vi "Transition Matrices_v1.vi"(6 "alpha":dbl, 8 "Tassign":dbl[](array[numeric])=[3.0, 4.0], 9 "theta":dbl=-0.6435 format="%#_13g", 10 "Rassign":dbl=1.0 format="%#_13g", 11 "R0":dbl) -> (1 "Translation Vector":dbl[](array[numeric]), 3 "Rotation Matrix":dbl[][](array[numeric]))   [LabVIEW 2010]
doc: "This file calculates the index-dependent rotation matrix and translation vector.\nReye is the eye radius, Rassign is the assigned radius, Tassign is the assigned translation vector.\nalpha is the scaling time-dependent parameter varys from 0 to 1."
uses:
  <vilib>/Analysis/NI_AALPro.lvlib
  <vilib>/Analysis/_algsub.llb/Real Vector Norm.vi
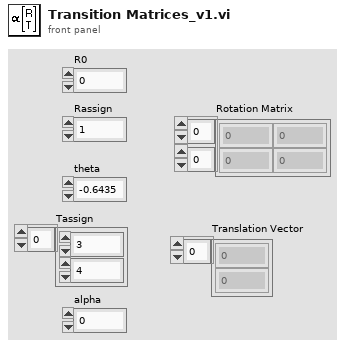
[diagram p1: front panel]
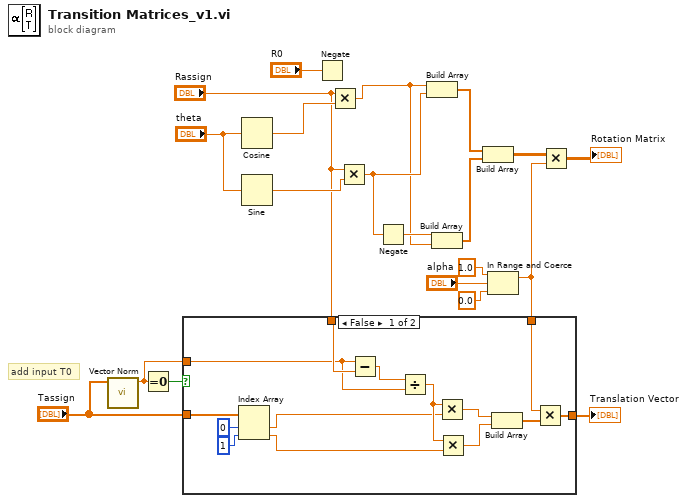
[diagram p0: block diagram]
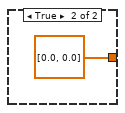
[diagram p2: hidden frame]
diagram:
  # "add input T0"
  n1 = call-poly <vilib>:"Vector Norm.vi"("Input Vector"="Tassign") -> ("norm"=w6:dbl)  [unwired: 9 in, 1 out]
  n2 = Equal To 0?(x=w6) -> (x = 0?=w4:bool)
  n3 = Cosine(x="theta") -> (cos(x)=w20:dbl)
  n4 = Sine(x="theta") -> (sin(x)=w19:dbl)
  n5 = Negate(x="R0") -> ()  [unwired: 1 out]
  n6 = Multiply(x="Rassign", y=w20) -> (x*y=w1:dbl)
  n7 = Multiply(x="Rassign", y=w19) -> (x*y=w17:dbl)
  n8 = Negate(x=w17) -> (-x=w16:dbl)
  n9 = Build Array(w1, w17) -> (w15:dbl[])
  n10 = Build Array(w16, w1) -> (w14:dbl[])
  n11 = Build Array(w15, w14) -> (w13:dbl[][])
  n12 = In Range and Coerce(upper limit=1.0, x="alpha", lower limit=0.0) -> (coerced(x)=w7:dbl)  [unwired: 1 out]
  n13 = case shown="False" w4 {
    tunnel: [w27 dbl[] [0.0, 0.0]] -> w11
    tunnel: w7 -> [w26 _]
    tunnel: "Rassign" -> [w25 _]
    tunnel: w6 -> [w24 _]
    tunnel: "Tassign" -> [w22 _]
    frame False {
      n14 = Index Array(array=w22, index #1=0 ("index"), index #2=1 ("index")) -> (element #1=w21:dbl, element #2=w23:dbl)
      n15 = Subtract(x=w24, y=w25) -> (x-y=w32:dbl)
      n16 = Divide(x=w32, y=w24) -> (x/y=w31:dbl)
      n17 = Multiply(x=w31, y=w21) -> (x*y=w30:dbl)
      n18 = Multiply(x=w31, y=w23) -> (x*y=w29:dbl)
      n19 = Build Array(w30, w29) -> (w28:dbl[])
      n20 = Multiply(x=w26, y=w28) -> (x*y=w27:dbl[])
    }
    frame True {
    }
  }
  "Translation Vector" <- w11
  n21 = Multiply(x=w13, y=w7) -> (x*y=→"Rotation Matrix":dbl[][])
